vi "I2C_Start_DAQ.vi"   [LabVIEW 2022 SP3]
panel:
  # "I2C_START"
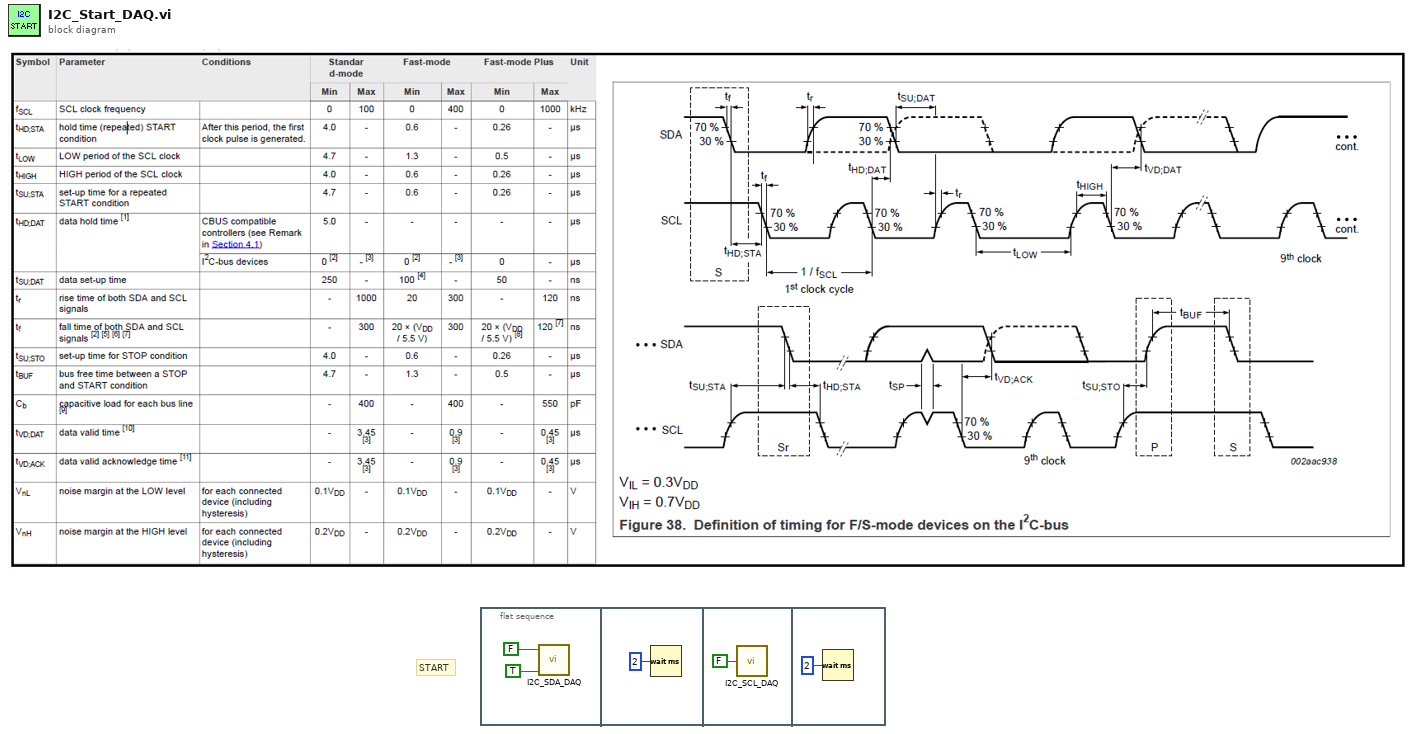
[diagram p0: block diagram]
diagram:
  # "START"
  n1 = flat-sequence {
    frame #0 {
      n2 = call "I2C_SDA_DAQ.vi"("Tx_or_Rx?"=TRUE, "Tx_Data"=FALSE) -> ()  [unwired: 1 in, 1 out]
    }
    frame #1 {
      n3 = Wait (ms)(milliseconds to wait=u32 2) -> ()  [unwired: 1 out]
    }
    frame #2 {
      n4 = call "I2C_SCL_DAQ.vi"("SCL_Data"=FALSE) -> ()  [unwired: 5 in]
    }
    frame #3 {
      n5 = Wait (ms)(milliseconds to wait=u32 2) -> ()  [unwired: 1 out]
    }
  }
